vi "Write_easy.vi"() -> ()   [LabVIEW 2023]
uses:
  <vilib>/numeric/Random Number (Range) U64.vi
  <vilib>/numeric/sub_Random U32.vi
  <vilib>/Utility/file.llb/Write Delimited Spreadsheet (I64).vi
panel:
  out "Numeric":i32
  out "path":path
  out "appended path":path
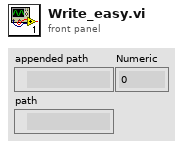
[diagram p1: front panel]
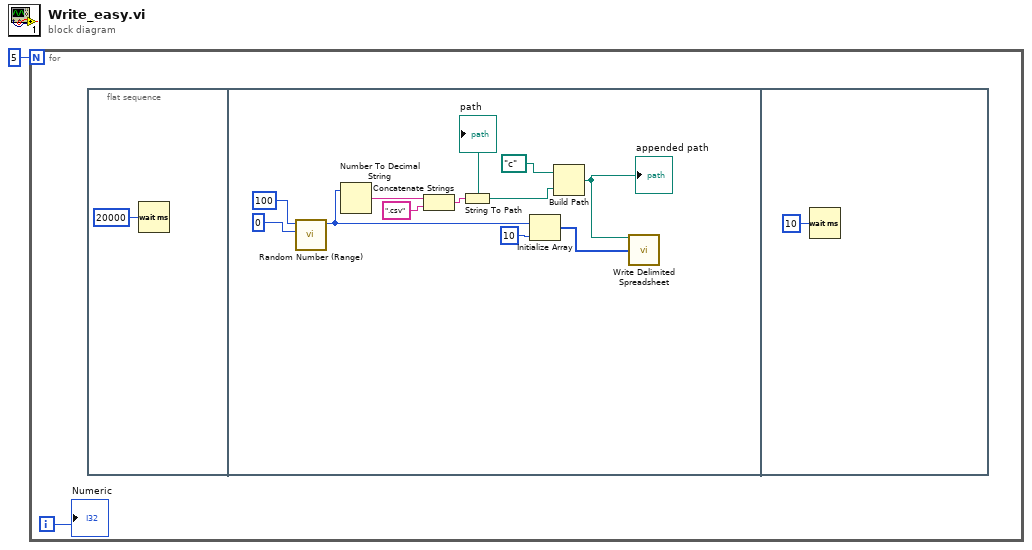
[diagram p0: block diagram]
diagram:
  n1 = for {
    N: 5 -> [_]
    i -> [w2]
    n2 = flat-sequence {
      frame #0 {
        n3 = Wait (ms)(milliseconds to wait=u32 20000) -> ()  [unwired: 1 out]
      }
      frame #1 {
        n4 = call-poly <vilib>:"Random Number (Range).vi"("lower bound (0)"=u64 0, "upper bound (100)"=u64 100) -> ("number"=w10:u64)  [unwired: 9 in]
        n5 = Number To Decimal String(number=w10) -> (decimal integer string=w8:string)  [unwired: 1 in]
        n6 = Concatenate Strings(w8, ".csv") -> (w7:string)
        n7 = String To Path(string=w7) -> (path=w4:path)
        "path" <- w4
        n8 = Initialize Array(w10, 10 ("dimension size")) -> (w14:u64[])
        n9 = Build Path(base path=path "c:/" ("file path (dialog if empty)"), name or relative path=w4) -> (appended path=w6:path)
        "appended path" <- w6
        n10 = call-poly <vilib>:"Write Delimited Spreadsheet.vi"("file path (dialog if empty)"=w6, "1D data"=w14) -> ()  [unwired: 12 in, 2 out]
      }
      frame #2 {
        n11 = Wait (ms)(milliseconds to wait=u32 10) -> ()  [unwired: 1 out]
      }
    }
    "Numeric" <- w2
  }
